vi "Generate_Report_NEW.vi"(0 "Max Voltage":dbl, 1 "Test Part":bool, 3 "Test Voltages (in)":dbl[](array[numeric])=[0.0, 0.1, 0.2, 0.3, 0.4, 0.5, 0.7, 1.0, 2.0, 3.0, 4.0, 5.0, 7.0, 10.0, 20.0, 30.0, 40.0, 50.0, 70.0, 100.0, 200.0], 5 "Min Voltage":dbl, 6 "Bi-directional Zener?":bool=TRUE, 8 "Chart Voltage Generation Method":u16(ring) items=["Linear", "Crude Semi-Log (Short)", "Crude Semi-Log (Long)", "Bi-directional Crude Semi-Log (Short)", "Bi-directional Crude Semi-Log (Long)"], 9 "Next Part":i32=17, 10 "Polarity for Max Voltage":u16(ring) items=["Positive", "Negative"], 11 "error in (no error)":errorcluster, 13 "Stop":bool) -> (2 "Test Voltages Chosen":dbl[](array[numeric]), 4 "XY Graph":cluster{"X":dbl, "Y":dbl}[](graph), 14 "Array":dbl[](array[numeric]), 15 "error out":errorcluster)   [LabVIEW 2020]
uses:
  <vilib>/Utility/file.llb/Write Delimited Spreadsheet (DBL).vi
  <vilib>/Utility/file.llb/Write Delimited Spreadsheet (string).vi
panel:
  in  "Which Button?":T1(ring)=enum."Center Button"
  in  "Capacitance Results Temp Array":dbl[](array[numeric])
  in  "Retest":bool
  in  "Default":i32=17
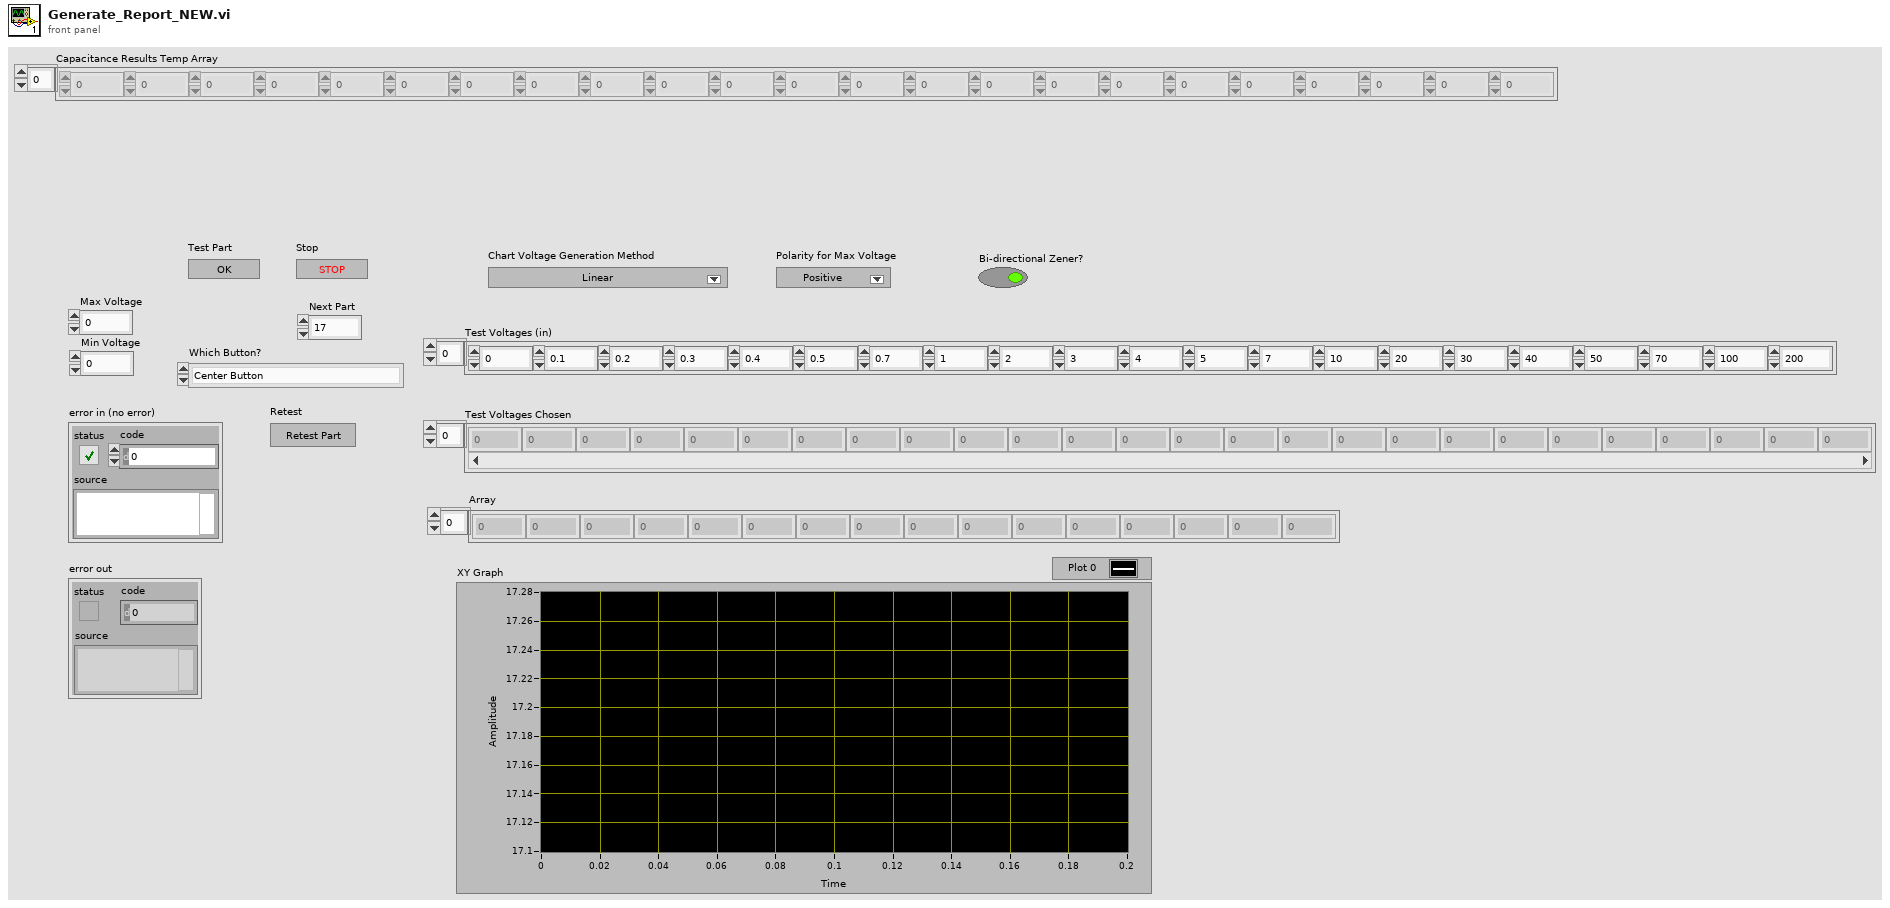
[diagram p1: front panel]
types:
  T1 = enum16{"Left Button", "Center Button", "Right Button", "Window Close"}
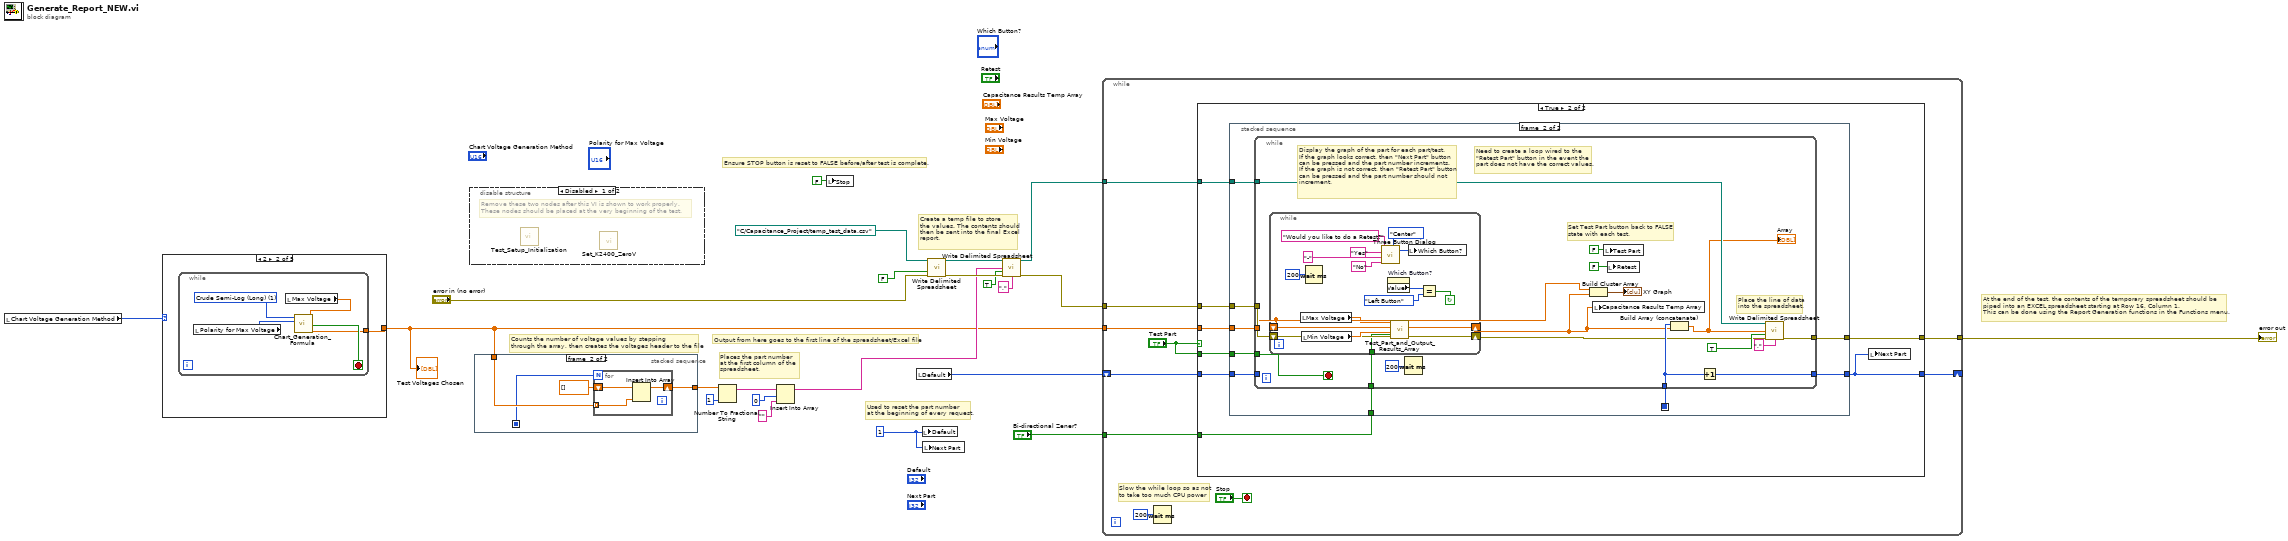
[diagram p0: block diagram]
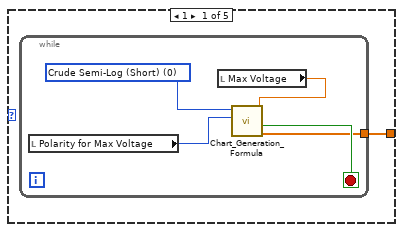
[diagram p3: hidden frame]
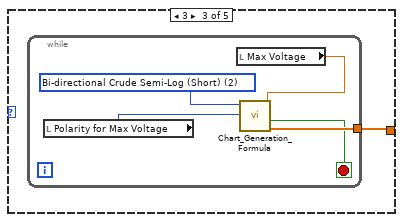
[diagram p4: hidden frame]
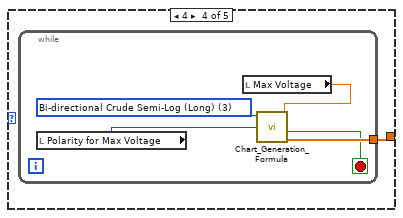
[diagram p5: hidden frame]
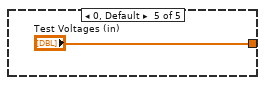
[diagram p6: hidden frame]
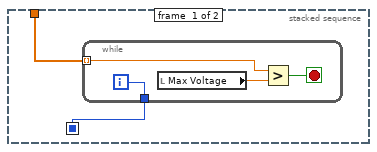
[diagram p7: hidden frame]
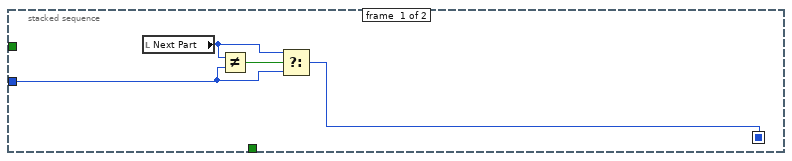
[diagram p9: hidden frame]
diagram:
  w16 = 1 ("New Part Number")
  # "At the end of the test, the contents of the temporary spreadsheet should be\npiped into an EXCEL spreadsheet starting at Row 16, Column 1. \nThis can be done using the Report Generation functions in the Functions menu."
  # "Ensure STOP button is reset to FALSE before/after test is complete."
  # "Places the part number\nat the first column of the \nspreadsheet."
  # "Used to reset the part number\nat the beginning of every request."
  # "Create a temp file to store\nthe values. The contents should\nthen be sent into the final Excel\nreport."
  # "Output from here goes to the first line of the spreadsheet/Excel file"
  # "Counts the number of voltage values by stepping\nthrough the array, then creates the voltages header to the file"
  n1 = local read "Chart Voltage Generation Method"() -> (w1:u16)
  n2 = case shown="2" w1 {
    tunnel: [w23 w29 w35 w41 "Test Voltages (in)"] -> w5
    frame 1 {
      n3 = while {
        tunnel: [w24] -> w23
        stop <- w25 stop-if-true
        w26 = u16 0 items=[" Crude Semi-Log (Short)", "Crude Semi-Log (Long)", "Bi-directional Crude Semi-Log (Short)", "Bi-directional Crude Semi-Log (Long)"] ("Type of Chart")
        n4 = local read "Polarity for Max Voltage"() -> (w28:u16)
        n5 = local read "Max Voltage"() -> (w27:dbl)
        n6 = call "Chart_Generation_Formula.vi"("Max Voltage"=w27, "Polarity for Max Voltage"=w28, "Type of Chart"=w26) -> ("Result - Test Voltages Array"=w24:dbl[], "~~ FINISH ~~"=w25:bool)  [unwired: 7 in]
      }
    }
    frame 2 {
      n7 = while {
        tunnel: [w30] -> w29
        stop <- w31 stop-if-true
        w32 = u16 1 items=[" Crude Semi-Log (Short)", "Crude Semi-Log (Long)", "Bi-directional Crude Semi-Log (Short)", "Bi-directional Crude Semi-Log (Long)"] ("Type of Chart")
        n8 = local read "Polarity for Max Voltage"() -> (w34:u16)
        n9 = local read "Max Voltage"() -> (w33:dbl)
        n10 = call "Chart_Generation_Formula.vi"("Max Voltage"=w33, "Polarity for Max Voltage"=w34, "Type of Chart"=w32) -> ("Result - Test Voltages Array"=w30:dbl[], "~~ FINISH ~~"=w31:bool)  [unwired: 7 in]
      }
    }
    frame 3 {
      n11 = while {
        tunnel: [w39] -> w35
        stop <- w38 stop-if-true
        w36 = u16 2 items=[" Crude Semi-Log (Short)", "Crude Semi-Log (Long)", "Bi-directional Crude Semi-Log (Short)", "Bi-directional Crude Semi-Log (Long)"] ("Type of Chart")
        n12 = local read "Polarity for Max Voltage"() -> (w37:u16)
        n13 = local read "Max Voltage"() -> (w40:dbl)
        n14 = call "Chart_Generation_Formula.vi"("Max Voltage"=w40, "Polarity for Max Voltage"=w37, "Type of Chart"=w36) -> ("Result - Test Voltages Array"=w39:dbl[], "~~ FINISH ~~"=w38:bool)  [unwired: 7 in]
      }
    }
    frame 4 {
      n15 = while {
        tunnel: [w44] -> w41
        stop <- w43 stop-if-true
        w42 = u16 3 items=[" Crude Semi-Log (Short)", "Crude Semi-Log (Long)", "Bi-directional Crude Semi-Log (Short)", "Bi-directional Crude Semi-Log (Long)"] ("Type of Chart")
        n16 = local read "Polarity for Max Voltage"() -> (w46:u16)
        n17 = local read "Max Voltage"() -> (w45:dbl)
        n18 = call "Chart_Generation_Formula.vi"("Max Voltage"=w45, "Polarity for Max Voltage"=w46, "Type of Chart"=w42) -> ("Result - Test Voltages Array"=w44:dbl[], "~~ FINISH ~~"=w43:bool)  [unwired: 7 in]
      }
    }
    frame 0, Default {
    }
  }
  "Test Voltages Chosen" <- w5
  n19 = disable-structure shown="Disabled" {
    frame Disabled {
      # "Remove these two nodes after this VI is shown to work properly.\nThese nodes should be placed at the very beginning of the test."
      n20 = call "Test_Setup_Initialization.vi"() -> ()  [unwired: 11 in, 1 out]
      n21 = call "Set_K2400_ZeroV.vi"() -> ()  [unwired: 11 in, 1 out]
    }
    frame Enabled {
    }
  }
  n22 = stacked-sequence {
    seq-local: [w48 _] -> [_ w55]
    tunnel: w5 -> [w49 w56]
    tunnel: [_ w57] -> w18
    frame #0 {
      n23 = while {
        tunnel: w49 -> [w51] mode=indexing
        tunnel: [w50] -> w48
        i -> [w50]
        stop <- w52 stop-if-true
        n24 = local read "Max Voltage"() -> (w53:dbl)
        n25 = Greater?(x=w51, y=w53) -> (0:w52:bool)
      }
    }
    frame #1 {
      n26 = for {
        N: w55 -> [_]
        tunnel: w56 -> [w60] mode=indexing
        shift-right: [w58] -> w57
        shift-left: dbl[] [] -> [w59]
        n27 = Insert Into Array(array=w59, new element=w60) -> (w58:dbl[])  [unwired: 1 in]
      }
    }
  }
  n28 = Number To Fractional String(number=w18, precision (6)=i16 1) -> (F-format string=w21:string[])  [unwired: 2 in]
  n29 = Insert Into Array(array=w21, index=0, new element="" ("new element/subarray")) -> (w9:string[])
  n30 = local write "Stop"(FALSE ("Stop")) -> ()
  n31 = local read "Default"() -> (w17:i32)
  n32 = local write "Default"(w16) -> ()
  n33 = local write "Next Part"(w16) -> ()
  n34 = call-poly <vilib>:"Write Delimited Spreadsheet.vi"("file path (dialog if empty)"=path "C:/Capacitance_Project/temp_test_data.csv", "append to file? (new file:F)"=FALSE, "error in (no error)"="error in (no error)") -> ("new file path (Not A Path if cancelled)"=w13:path, "error out"=w11:errorcluster)  [unwired: 11 in]
  n35 = call-poly <vilib>:"Write Delimited Spreadsheet.vi"("file path (dialog if empty)"=w13, "1D data"=w9, "append to file? (new file:F)"=TRUE, "error in (no error)"=w11, "delimiter (\\t)"="," ("delimiter (\\t)")) -> ("new file path (Not A Path if cancelled)"=w12:path, "error out"=w10:errorcluster)  [unwired: 9 in]
  n36 = while {
    tunnel: w5 -> [w70]
    shift-right: [w65] -> _
    shift-left: w17 -> [w66]
    tunnel: [w64] -> w4
    tunnel: w10 -> [w63]
    tunnel: "Bi-directional Zener?" -> [w62]
    tunnel: w12 -> [w61]
    stop <- "Stop" stop-if-true
    # "Slow the while loop so as not\nto take too much CPU power"
    n37 = Wait (ms)(milliseconds to wait=u32 200) -> ()  [unwired: 1 out]
    n38 = case shown="True" "Test Part" {
      tunnel: w70 -> [_ w79]
      tunnel: "Test Part" -> [_ w80]
      tunnel: w66 -> [w72 w76]
      tunnel: [w72 w75] -> w65
      tunnel: [w71 w78] -> w64
      tunnel: w63 -> [w71 w77]
      tunnel: w62 -> [_ w74]
      tunnel: w61 -> [_ w73]
      frame False {
      }
      frame True {
        n39 = stacked-sequence {
          seq-local: [w82 _] -> [_ w87]
          tunnel: [_ w93] -> w75
          tunnel: w80 -> [_ w92]
          tunnel: w79 -> [_ w91]
          tunnel: [_ w90] -> w78
          tunnel: w77 -> [_ w89]
          tunnel: w76 -> [w81 w88]
          tunnel: w74 -> [_ w86]
          tunnel: w73 -> [_ w85]
          frame #0 {
            n40 = local read "Next Part"() -> (w84:i32)
            n41 = Not Equal?(x=w84, y=w81) -> (x != y?=w83:bool)
            n42 = Select(t=w84, s=w83, f=w81) -> (s? t:f=w82:i32)
          }
          frame #1 {
            n43 = while {
              tunnel: w91 -> [w100]
              tunnel: w92 -> [w94]
              tunnel: w88 -> [_]
              tunnel: [w108] -> w93
              tunnel: [w103] -> w90
              tunnel: w89 -> [w110]
              tunnel: w87 -> [w109]
              tunnel: w86 -> [w107]
              tunnel: w85 -> [w106]
              stop <- w94 stop-if-true
              # "Set Test Part button back to FALSE\nstate with each test."
              # "Place the line of data\ninto the spreadsheet."
              # "Display the graph of the part for each part/test.\nIf the graph looks correct, then \"Next Part\" button\ncan be pressed and the part number increments.\nIf the graph is not correct, then \"Retest Part\" button\ncan be pressed and the part number should not\nincrement."
              # "Need to create a loop wired to the \n\"Retest Part\" button in the event the \npart does not have the correct values."
              n44 = while {
                tunnel: w107 -> [w124]
                shift-right: [w123] -> w104
                shift-left: w110 -> [w125]
                shift-right: [w121] -> w99
                shift-left: w100 -> [w122]
                stop <- w112 continue-if-true
                n45 = local read "Max Voltage"() -> (w127:dbl)
                n46 = local read "Min Voltage"() -> (w126:dbl)
                n47 = Wait (ms)(milliseconds to wait=u32 200) -> ()  [unwired: 1 out]
                n48 = call <vilib>:"Three Button Dialog.vi"("Justify Message (Left)"=enum16{"Left", "Center", "Right"}."Center", "Right Button Text (\"Cancel\")"="No" ("Right Button Text (\"Cancel\")"), "Center Button Text (\"No\")"="-" ("Center Button Text (\"No\")"), "Left Button Text (\"Yes\")"="Yes" ("Left Button Text (\"Yes\")"), "message"="Would you like to do a Retest?") -> ("Which Button?"=w116:T1)  [unwired: 6 in]
                n49 = property on="Which Button?" class="Enum (strict)"() -> ("Value"=w114:T1)  [unwired: 2 in, 2 out]
                n50 = call "Test_Part_and_Output_Results_Array.vi"("Bi-directional Zener?"=w124, "error in"=w125, "Min Voltage"=w126, "Input Voltages Array"=w122, "Max Voltage"=w127) -> ("error out"=w123:errorcluster, "Capacitance Results Array"=w121:dbl[])  [unwired: 3 in, 2 out]
                n51 = local write "Which Button?"(w116) -> ()
                n52 = Equal?(x=w114, y=T1."Left Button" ("Which Button?")) -> (x = y?=w112:bool)
              }
              n53 = Wait (ms)(milliseconds to wait=u32 200) -> ()  [unwired: 1 out]
              n54 = Build Cluster Array ("Index & Bundle Cluster Array")(w100, w99) -> (→"XY Graph":cluster{dbl, dbl}[])
              n55 = local write "Capacitance Results Temp Array"(w99) -> ()
              n56 = local write "Test Part"(FALSE ("Test Part")) -> ()
              n57 = local write "Retest"(FALSE ("Test Part")) -> ()
              n58 = Build Array (concatenate)(w109, w99) -> (w101:dbl[])
              "Array" <- w101
              n59 = Increment(x=w109) -> (x+1=w108:i32)
              n60 = call-poly <vilib>:"Write Delimited Spreadsheet.vi"("file path (dialog if empty)"=w106, "1D data"=w101, "append to file? (new file:F)"=TRUE, "error in (no error)"=w104, "delimiter (\\t)"="," ("delimiter (\\t)")) -> ("error out"=w103:errorcluster)  [unwired: 9 in, 1 out]
            }
          }
        }
        n61 = local write "Next Part"(w75) -> ()
      }
    }
  }
  "error out" <- w4
